vi "get channels.vi"(11 "tag select module configuration in":refnum<class "Table Test configuration.lvclass">) -> (2 "channels":refnum<class "TBM channel.lvclass">[](array[class]), 3 "tag select module configuration out":refnum<class "Table Test configuration.lvclass">)   [LabVIEW 2013, in "Table Test configuration.lvclass"]
uses:
  Table Test configuration.lvclass
  <vilib>/NI/Tag Bus Module Framework/channel/TBM channel.lvclass
  Table Test configuration.lvclass/Table Test configuration.ctl
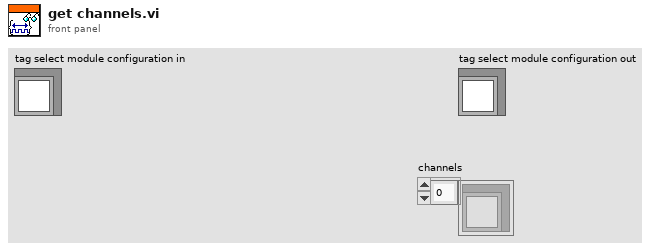
[diagram p1: front panel]
types:
  T1 = typedef "Table Test configuration.lvclass/tag select configuration.ctl" = cluster{"tag select name":string, "data type":T2, "output":refnum<class "TBM channel.lvclass">, "select":refnum<class "TBM channel.lvclass">, "input channels":refnum<class "TBM channel.lvclass">[]}
  T2 = typedef "tag bus.lvlib/tag descriptor.lvclass/Data Type.ctl" = enum16{"Double", "Single", "I64", "I32", "I16", "I8", "U64", "U32", "U16", "U8", "Boolean", "String", "Array of Double", "Array of Single", "Array of I64", "Array of I32", "Array of I16", "Array of I8", "Array of U64", "Array of U32", "Array of U16", "Array of U8", "Array of Boolean", "Array of String"}
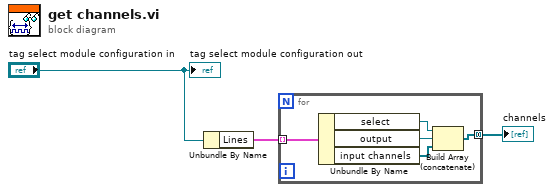
[diagram p0: block diagram]
diagram:
  n1 = Unbundle By Name("tag select module configuration in") -> ("Lines"=w2:T1[])
  n2 = for {
    tunnel: w2 -> [w7] mode=indexing
    tunnel: [w8] -> w1 mode=concatenating
    n3 = Unbundle By Name(w7) -> ("select"=w5:refnum<class "TBM channel.lvclass">, "output"=w6:refnum<class "TBM channel.lvclass">, "input channels"=w4:refnum<class "TBM channel.lvclass">[])
    n4 = Build Array (concatenate)(w5, w6, w4) -> (w8:refnum<class "TBM channel.lvclass">[])
  }
  "channels" <- w1
  "tag select module configuration out" <- "tag select module configuration in"
